vi "Broadcast Agitator Settings.vi"(8 "error in (no error)":errorcluster, 10 "Message Queues":T5, 11 "Agitator Module Config":T1={"GUID"="", "Drop Coords"={"Horizontal"=0, "Vertical"=0}, "Process Name"="", "User name"="", "Queue Name"="", "Settings"={"Cycle Period"=500.0, "Agitator Type"="", "Setpoint (µm)"=0.0, "IKA EUROSTAR Settings"={"VISA resource name"="", "Simulated?"=FALSE}}, "Load Count"=0}) -> (0 "error out":errorcluster)   [LabVIEW 2018, in "Agitator Module.lvlib"]
uses:
  Agitator Module.lvlib
  Agitator Message Queues.ctl
  support/Message Queue/Message Cluster.ctl
  Controls/Agitator Module Config Cluster.ctl
  <vilib>/Utility/miscctls.llb/LVPoint32TypeDef.ctl
  Controls/Agitator Module Settings Cluster.ctl
  IKA EUROSTAR/IKA EUROSTAR Settings.ctl
  support/Message Queue/Enqueue Message (Single).vi
  support/Message Queue/Message Queue.lvlib
  IKA EUROSTAR/IKA EUROSTAR.lvlib
panel:
  # "Agitator Settings"
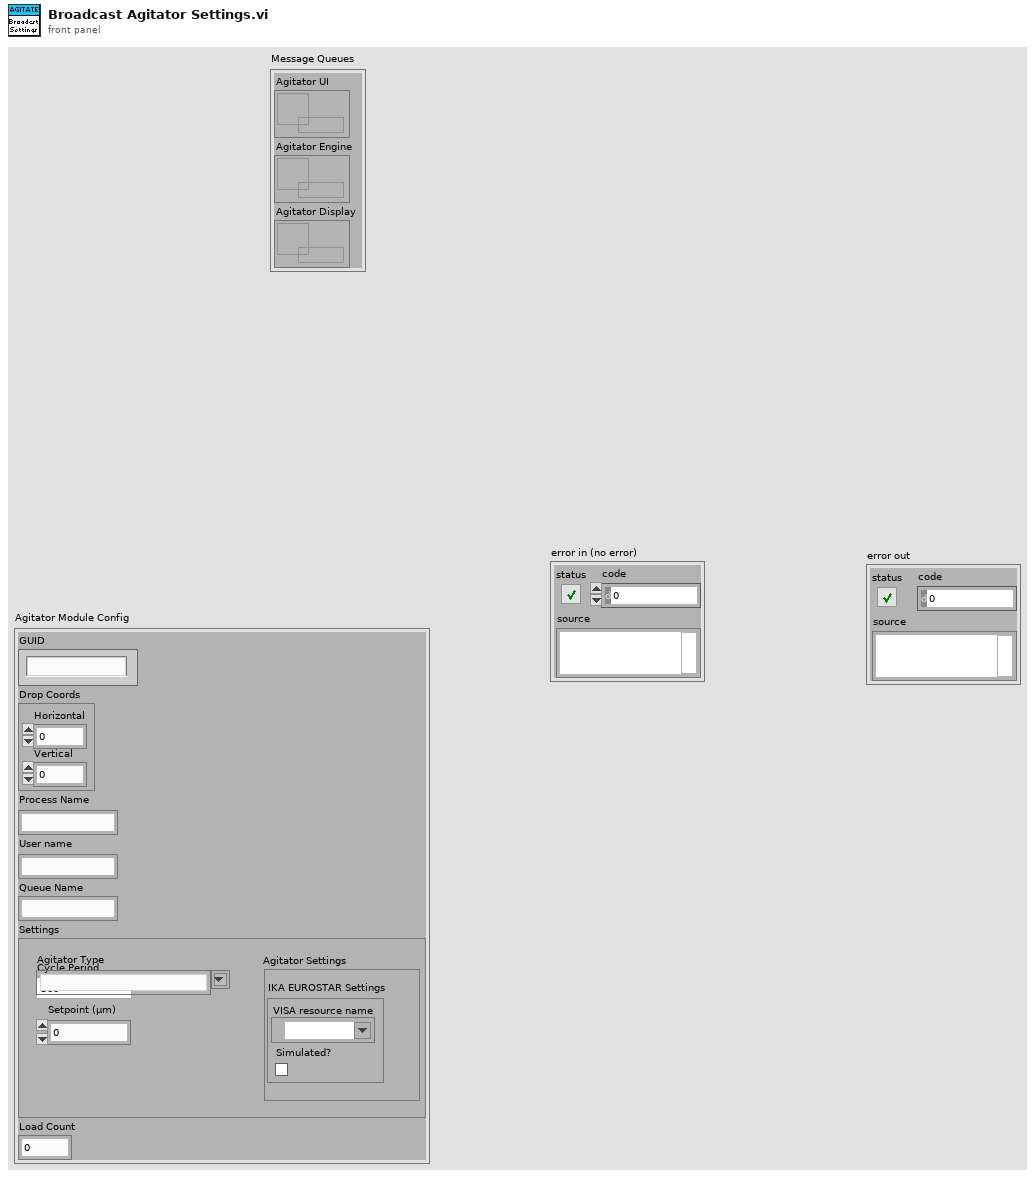
[diagram p1: front panel]
types:
  T1 = typedef "Agitator Module.lvlib/Agitator Module Config Cluster.ctl" = cluster{"GUID":string, "Drop Coords":T2, "Process Name":string, "User name":string, "Queue Name":string, "Settings":T3, "Load Count":i32}
  T2 = typedef "LVPoint32TypeDef.ctl" = cluster{"Horizontal":i32, "Vertical":i32}
  T3 = typedef "Agitator Module.lvlib/Agitator Module Settings Cluster.ctl" = cluster{"Cycle Period":dbl, "Agitator Type":string, "Setpoint (µm)":dbl, "IKA EUROSTAR Settings":T4}
  T4 = typedef "IKA EUROSTAR.lvlib/IKA EUROSTAR Settings.ctl" = cluster{"VISA resource name":refnum<visa-resource-name>, "Simulated?":bool}
  T5 = typedef "Agitator Module.lvlib/Agitator Message Queues.ctl" = cluster{"Agitator UI":refnum<queue>, "Agitator Engine":refnum<queue>, "Agitator Display":refnum<queue>}
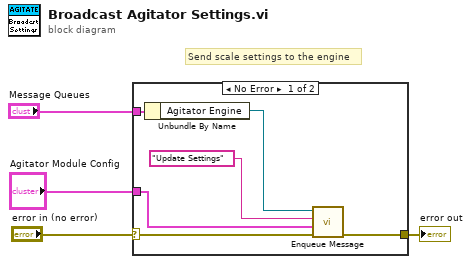
[diagram p0: block diagram]
diagram:
  # "Send scale settings to the engine"
  n1 = case shown="No Error" "error in (no error)" {
    selector: "error in (no error)" -> [w6 w11]
    tunnel: [w5 w11] -> w2
    tunnel: "Agitator Module Config" -> [w8 _]
    tunnel: "Message Queues" -> [w10 _]
    frame No Error {
      n2 = Unbundle By Name(w10) -> ("Agitator Engine"=w9:refnum<queue>)
      n3 = call-poly "Enqueue Message.vi"("error in (no error)"=w6, "Message Data"=w8, "Message"="Update Settings", "Message Queue"=w9) -> ("error out"=w5:errorcluster)  [unwired: 6 in, 1 out]
    }
    frame Error {
    }
  }
  "error out" <- w2
